vi "Configure Frequency.vi"(7 "Channel (1:Channel 1)":i32(ring)=1 items=["Channel 1"=1, "Channel 2"=2, "Channel 3"=3], 8 "error in (no error)":errorcluster, 9 "Frequency Estimate (10E+6 Hz)":dbl=10000000.0 format="%^#_6g", 11 "VISA resource name":refnum<visa-resource-name>) -> (0 "error out":errorcluster, 3 "VISA resource name out":refnum<visa-resource-name>)   [LabVIEW 2018, in "Counter.lvlib" / "PICOTEST U62XXA series.lvlib"]
doc: "Configures the settings required for a Frequecy measurement.\n\n<B>Note:</B>\n\nThe measurement arming is coupled to Auto. Arming can be changed by calling any of the Arming VIs. The measurement channel has auto-trigger enabled at 50% with a positive slope."
uses:
  PICOTEST U62XXA series.lvlib
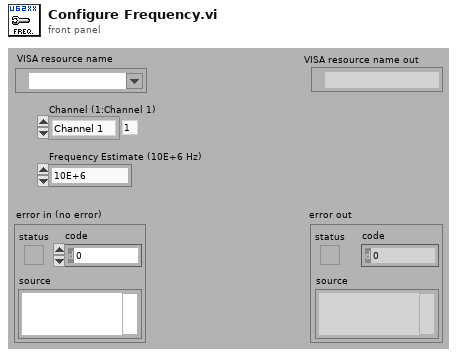
[diagram p1: front panel]
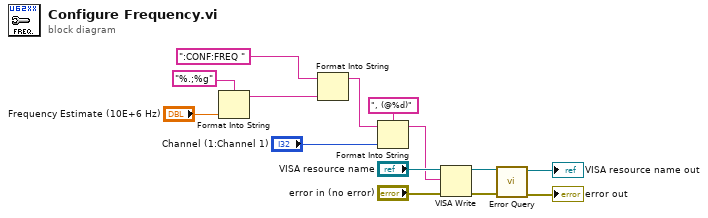
[diagram p0: block diagram]
diagram:
  n1 = Format Into String(format string="%.;%g", "Frequency Estimate (10E+6 Hz)") -> (resulting string=w3:string)  [unwired: 2 in, 1 out]
  n2 = Format Into String(initial string=":CONF:FREQ " ("string (\"\")"), w3) -> (resulting string=w2:string)  [unwired: 2 in, 1 out]
  n3 = Format Into String(format string=", (@%d)", initial string=w2, "Channel (1:Channel 1)") -> (resulting string=w9:string)  [unwired: 1 in, 1 out]
  n4 = VISA Write(VISA resource name="VISA resource name", write buffer=w9, error in (no error)="error in (no error)") -> (VISA resource name out=w8:refnum<visa-resource-name>, error out=w6:errorcluster)  [unwired: 1 out]
  n5 = call "Error Query.vi"("error in (no error)"=w6, "VISA resource name"=w8) -> ("error out"=→"error out":errorcluster, "VISA resource name out"=→"VISA resource name out":refnum<visa-resource-name>)  [unwired: 6 in, 2 out]
